vi "Find Last Number.vi"(11 "String in":string) -> (3 "first number":string)   [LabVIEW 2022 SP3]
uses:
  <vilib>/regexp/Match Regular Expression.xnode
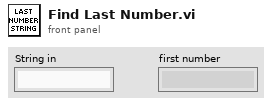
[diagram p1: front panel]
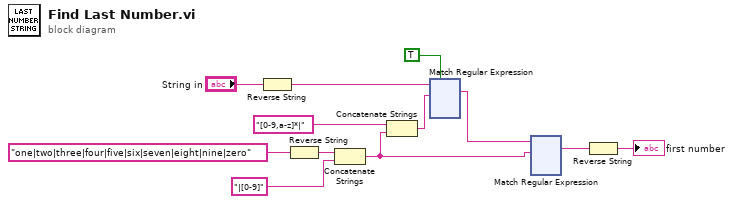
[diagram p0: block diagram]
diagram:
  n1 = Reverse String(1:"String in") -> (0:w9:string)
  n2 = Reverse String(1:"one|two|three|four|five|six|seven|eight|nine|zero" ("format string")) -> (0:w8:string)
  n3 = Concatenate Strings(w8, "|[0-9]" ("format string")) -> (w3:string)
  n4 = Concatenate Strings("[0-9,a-z]*|" ("format string"), w3) -> (w10:string)
  n5 = xnode "Match Regular Expression"("input string"=w9, "regular expression"=w10, "ignore case? (F)"=TRUE) -> ("whole match"=w4:string)  [unwired: 3 in, 4 out]
  n6 = xnode "Match Regular Expression"("input string"=w4, "regular expression"=w3) -> ("whole match"=w7:string)  [unwired: 4 in, 4 out]
  n7 = Reverse String(1:w7) -> (0:→"first number":string)
